vi "Swarm Method.vi"() -> ()   [LabVIEW 2014]
uses:
  <vilib>/Analysis/NI_AALPro.lvlib
  <vilib>/Analysis/baseanly.llb/Matrix Type of Inverse Matrix.ctl
  <vilib>/Analysis/NI_AALBase.lvlib
  <vilib>/Analysis/7linalg.llb/Solve Linear Equations (single right hand).vi
  Anchor/Anchor.lvclass
panel:
  in  "AnchorsArray":refnum<class "Anchor.lvclass">[](array[class])
  in  "Max bereik":dbl
  in  "d tags anchors":dbl[][](array[numeric])
  out "tag 3":i32
  in  "d tags onderling":dbl[](array[numeric])
  out "Solution Vector":dbl[](array[numeric]) format="%.2f"
  in  "Werkpunten":cluster{"a":dbl, "b":dbl}[](array[cluster])
  in  "# tags":i32=22
  out "tag 2":i32
  out "Tag 1":i32
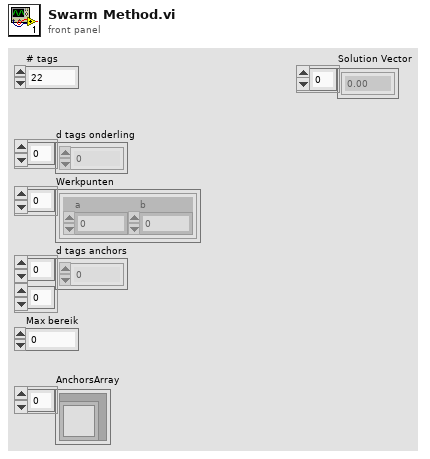
[diagram p1: front panel]
types:
  T1 = typedef "NI_AALBase.lvlib/Matrix Type of Inverse Matrix.ctl" = enum32{"General", "Positive Definite", "Lower Triangular", "Upper Triangular"}
  T2 = cluster{"Tag.lvclass":refnum<class "Tag.lvclass">, "Distance":dbl}[]
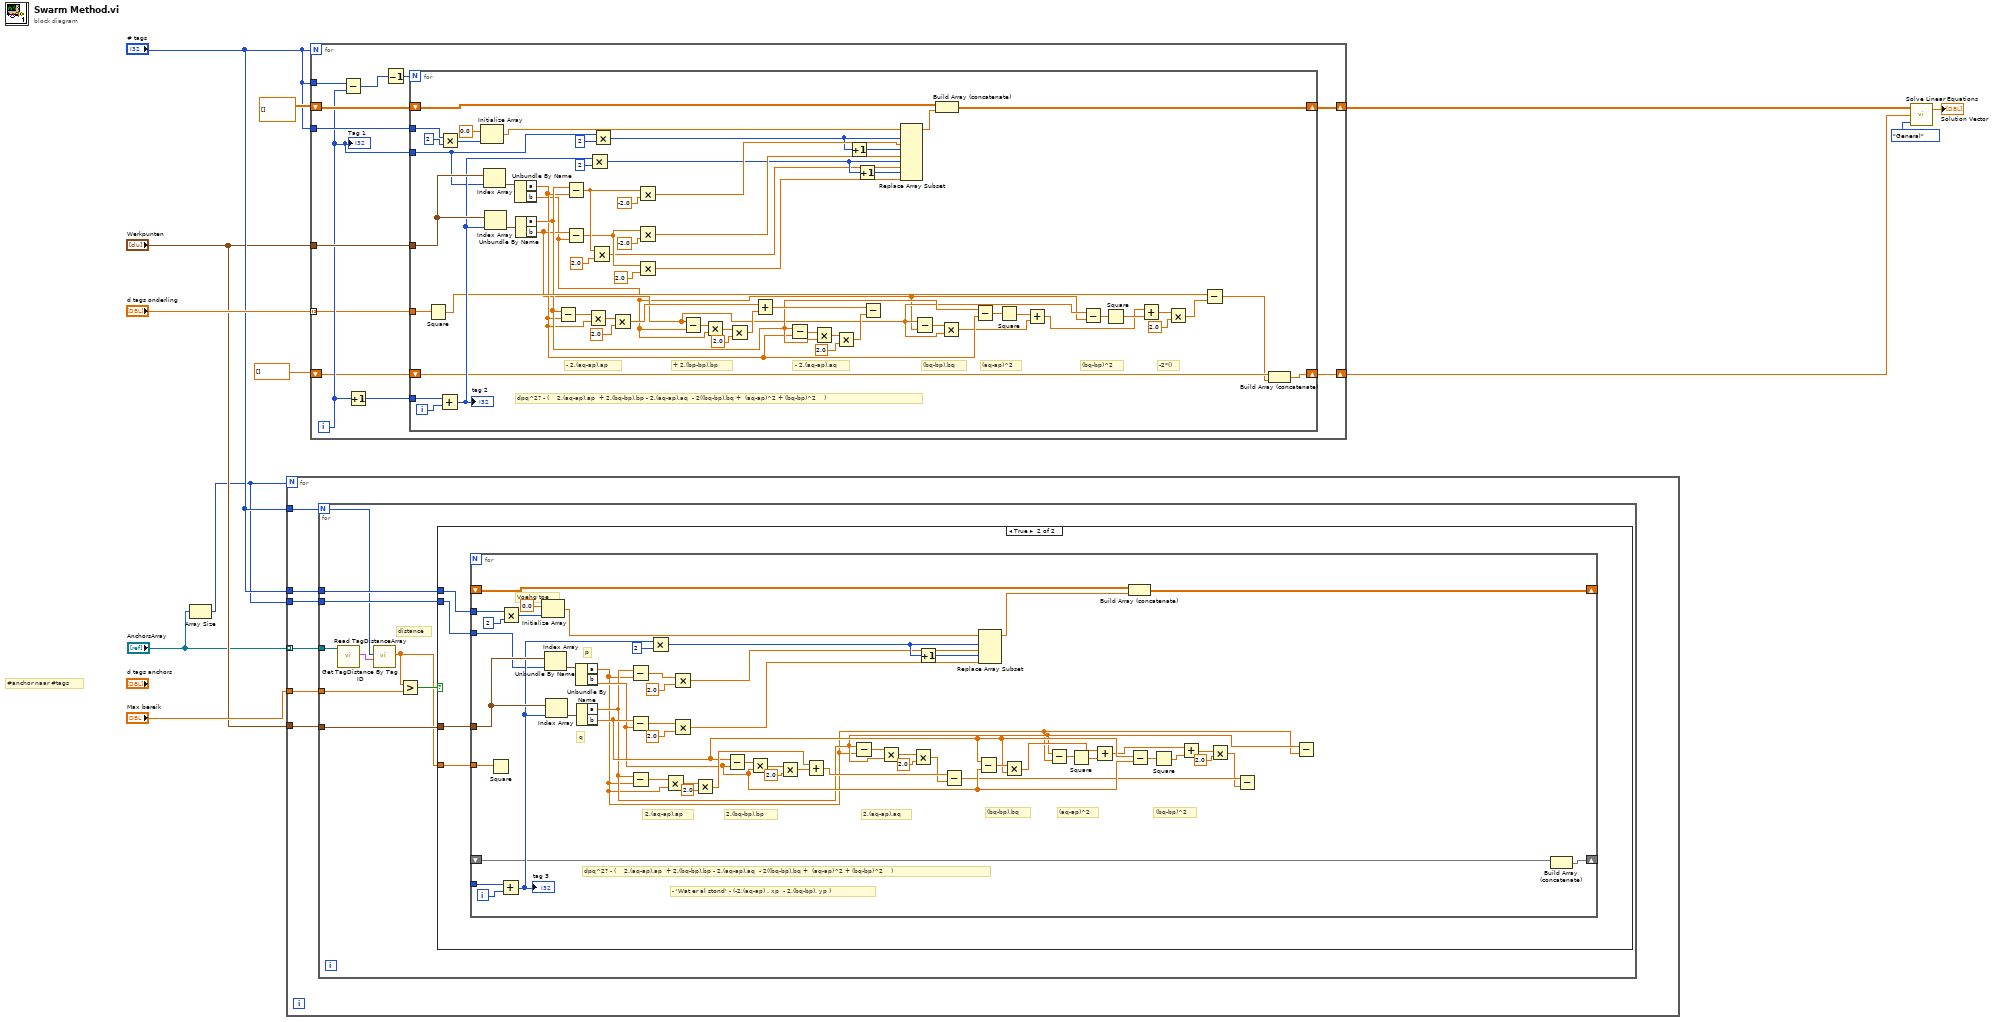
[diagram p0: block diagram]
diagram:
  # "#anchor naar #tags"
  n1 = Array Size(array="AnchorsArray") -> (size(s)=w1:i32)
  n2 = for {
    N: w1 -> [_]
    tunnel: "# tags" -> [w16]
    tunnel: "Max bereik" -> [w18]
    tunnel: "Werkpunten" -> [w17]
    tunnel: "# tags" -> [w15]
    tunnel: w1 -> [w14]
    tunnel: "AnchorsArray" -> [w13] mode=indexing
    n3 = for {
      N: w16 -> [w20]
      tunnel: w18 -> [w26]
      tunnel: w17 -> [w25]
      tunnel: w14 -> [w24]
      tunnel: w15 -> [w23]
      tunnel: w13 -> [w22]
      # "distance"
      n4 = call-dynamic "Read TagDistanceArray.vi"("Anchor in"=w22) -> ("TagDistanceArray"=w21:T2)  [unwired: 8 in, 2 out]
      n5 = call "Get TagDistance By Tag ID.vi"("TagDistanceArray"=w21, "TagID"=w20) -> ("Distance"=w19:dbl)  [unwired: 9 in]
      n6 = Greater?(x=w19, y=w26) -> (0:w27:bool)
      n7 = case shown="True" w27 {
        tunnel: w25 -> [_ w31]
        tunnel: w24 -> [_ w30]
        tunnel: w23 -> [_ w29]
        tunnel: w19 -> [_ w28]
        frame False {
        }
        frame True {
          # "Voehg toe"
          n8 = for {
            tunnel: _ -> [w85]
            shift-right: [w84] -> _
            shift-left: _ -> [w78]
            tunnel: w29 -> [w80]
            tunnel: w31 -> [w75]
            tunnel: w30 -> [w62]
            shift-right: [w61] -> _
            shift-left: _ -> [w63]
            tunnel: w28 -> [w60]
            i -> [w86]
            # "(bq-bp)^2"
            # "(aq-ap)^2"
            # "(bq-bp).bq"
            # "2.(aq-ap).aq"
            # "2.(bq-bp).bp"
            # "2.(aq-ap).ap"
            # "q"
            # "p"
            # "-\t'Wat er al stond' - (-2.(aq-ap) . xp  - 2.(bq-bp). yp )"
            # "dpq^2? - (    2.(aq-ap).ap  + 2.(bq-bp).bp - 2.(aq-ap).aq  - 2((bq-bp).bq +  (aq-ap)^2 + (bq-bp)^2    )"
            n9 = Square(x=w60) -> ()  [unwired: 1 out]
            n10 = Add(x=w85, y=w86) -> (x+y=w72:i32)
            "tag 3" <- w72
            n11 = Multiply(x=w80, y=2) -> (x*y=w83:i32)
            n12 = Initialize Array(0.0 ("element"), w83) -> (w77:dbl[])
            n13 = Index Array(array=w75, index=w62) -> (element=w76:cluster{"a":dbl, "b":dbl})
            n14 = Index Array(array=w75, index=w72) -> (element=w74:cluster{"a":dbl, "b":dbl})
            n15 = Unbundle By Name(w76) -> ("a"=w32:dbl, "b"=w41:dbl)
            n16 = Unbundle By Name(w74) -> ("a"=w33:dbl, "b"=w42:dbl)
            n17 = Subtract(x=w33, y=w32) -> (x-y=w67:dbl)
            n18 = Subtract(x=w42, y=w41) -> (x-y=w66:dbl)
            n19 = Subtract(x=w33, y=w32) -> (x-y=w59:dbl)
            n20 = Multiply(x=w72, y=2) -> (x*y=w71:i32)
            n21 = Multiply(x=w59, y=w32) -> (x*y=w58:dbl)
            n22 = Multiply(x=w67, y=2.0) -> (x*y=w65:dbl)
            n23 = Multiply(x=w66, y=2.0) -> (x*y=w64:dbl)
            n24 = Multiply(x=w58, y=2.0) -> (x*y=w53:dbl)
            n25 = Subtract(x=w42, y=w41) -> (x-y=w56:dbl)
            n26 = Multiply(x=w56, y=w41) -> (x*y=w55:dbl)
            n27 = Multiply(x=w55, y=2.0) -> (x*y=w52:dbl)
            n28 = Add(x=w53, y=w52) -> (x+y=w48:dbl)
            n29 = Subtract(x=w33, y=w32) -> (x-y=w51:dbl)
            n30 = Multiply(x=w51, y=w33) -> (x*y=w50:dbl)
            n31 = Multiply(x=w50, y=2.0) -> (x*y=w47:dbl)
            n32 = Increment(x=w71) -> (x+1=w70:i32)
            n33 = Subtract(x=w48, y=w47) -> (x-y=w35:dbl)
            n34 = Subtract(x=w42, y=w41) -> (x-y=w46:dbl)
            n35 = Replace Array Subset(array=w77, new element #1=w65, index #1=w71, new element #2=w64, index #2=w70) -> (w79:dbl[])
            n36 = Multiply(x=w46, y=w42) -> (x*y=w44:dbl)
            n37 = Subtract(x=w33, y=w32) -> (x-y=w45:dbl)
            n38 = Square(x=w45) -> (x^2=w43:dbl)
            n39 = Add(x=w44, y=w43) -> (x+y=w39:dbl)
            n40 = Build Array (concatenate)(w78, w79) -> (w84:dbl[][])
            n41 = Subtract(x=w42, y=w41) -> (x-y=w40:dbl)
            n42 = Square(x=w40) -> (x^2=w38:dbl)
            n43 = Add(x=w39, y=w38) -> (x+y=w37:dbl)
            n44 = Multiply(x=w37, y=2.0) -> (x*y=w34:dbl)
            n45 = Subtract(x=w35, y=w34) -> ()  [unwired: 1 out]
            n46 = Subtract(x=w33, y=w32) -> ()  [unwired: 1 out]
            n47 = Build Array (concatenate)(w63) -> (w61:void[])  [unwired: 1 in]
          }
        }
      }
    }
  }
  n48 = for {
    N: "# tags" -> [_]
    tunnel: "# tags" -> [w98]
    shift-right: [w93] -> w11
    shift-left: dbl[][] [] -> [w94]
    tunnel: "# tags" -> [w92]
    tunnel: "Werkpunten" -> [w91]
    shift-right: [w89] -> w9
    shift-left: dbl[] [] -> [w88]
    tunnel: "d tags onderling" -> [w87] mode=indexing
    i -> [w90]
    n49 = Subtract(x=w98, y=w90) -> (x-y=w97:i32)
    n50 = Increment(x=w90) -> (x+1=w95:i32)
    n51 = Decrement(x=w97) -> (x-1=w96:i32)
    n52 = for {
      N: w96 -> [_]
      tunnel: w95 -> [w160]
      shift-right: [w159] -> w93
      shift-left: w94 -> [w153]
      tunnel: w92 -> [w155]
      tunnel: w91 -> [w150]
      tunnel: w90 -> [w130]
      shift-right: [w129] -> w89
      shift-left: w88 -> [w131]
      tunnel: w87 -> [w128]
      i -> [w161]
      # "-2*()"
      # "(bq-bp)^2"
      # "(aq-ap)^2"
      # "(bq-bp).bq"
      # "- 2.(aq-ap).aq"
      # "+ 2.(bp-bp).bp"
      # "- 2.(aq-ap).ap"
      # "dpq^2? - (    2.(aq-ap).ap  + 2.(bq-bp).bp - 2.(aq-ap).aq  - 2((bq-bp).bq +  (aq-ap)^2 + (bq-bp)^2    )"
      n53 = Square(x=w128) -> (x^2=w127:dbl)
      n54 = Add(x=w160, y=w161) -> (x+y=w140:i32)
      "tag 2" <- w140
      n55 = Multiply(x=w155, y=2) -> (x*y=w158:i32)
      n56 = Initialize Array(0.0 ("element"), w158) -> (w152:dbl[])
      n57 = Index Array(array=w150, index=w130) -> (element=w151:cluster{"a":dbl, "b":dbl})
      n58 = Index Array(array=w150, index=w140) -> (element=w149:cluster{"a":dbl, "b":dbl})
      n59 = Unbundle By Name(w151) -> ("a"=w111:dbl, "b"=w106:dbl)
      n60 = Unbundle By Name(w149) -> ("a"=w112:dbl, "b"=w107:dbl)
      n61 = Subtract(x=w112, y=w111) -> (x-y=w125:dbl)
      n62 = Subtract(x=w112, y=w111) -> (x-y=w135:dbl)
      n63 = Subtract(x=w107, y=w106) -> (x-y=w134:dbl)
      n64 = Multiply(x=w125, y=w111) -> (x*y=w124:dbl)
      n65 = Multiply(x=w140, y=2) -> (x*y=w139:i32)
      n66 = Multiply(x=w135, y=2.0) -> (x*y=w133:dbl)
      n67 = Multiply(x=w130, y=2) -> (x*y=w143:i32)
      n68 = Multiply(x=w124, y=2.0) -> (x*y=w123:dbl)
      n69 = Multiply(x=w135, y=-2.0) -> (x*y=w146:dbl)
      n70 = Multiply(x=w134, y=-2.0) -> (x*y=w144:dbl)
      n71 = Multiply(x=w134, y=2.0) -> (x*y=w132:dbl)
      n72 = Subtract(x=w107, y=w106) -> (x-y=w122:dbl)
      n73 = Multiply(x=w122, y=w106) -> (x*y=w121:dbl)
      n74 = Multiply(x=w121, y=2.0) -> (x*y=w119:dbl)
      n75 = Add(x=w123, y=w119) -> (x+y=w115:dbl)
      n76 = Subtract(x=w112, y=w111) -> (x-y=w118:dbl)
      n77 = Multiply(x=w118, y=w112) -> (x*y=w117:dbl)
      n78 = Multiply(x=w117, y=2.0) -> (x*y=w114:dbl)
      n79 = Increment(x=w143) -> (x+1=w142:i32)
      n80 = Increment(x=w139) -> (x+1=w138:i32)
      n81 = Subtract(x=w115, y=w114) -> ()  [unwired: 1 out]
      n82 = Replace Array Subset(array=w152, new element #1=w146, index #1=w143, new element #2=w144, index #2=w142, new element #3=w133, index #3=w139, new element #4=w132, index #4=w138) -> (w154:dbl[])
      n83 = Subtract(x=w107, y=w106) -> (x-y=w113:dbl)
      n84 = Build Array (concatenate)(w153, w154) -> (w159:dbl[][])
      n85 = Multiply(x=w113, y=w107) -> (x*y=w108:dbl)
      n86 = Subtract(x=w112, y=w111) -> (x-y=w110:dbl)
      n87 = Square(x=w110) -> (x^2=w109:dbl)
      n88 = Add(x=w109, y=w108) -> (x+y=w103:dbl)
      n89 = Subtract(x=w107, y=w106) -> (x-y=w105:dbl)
      n90 = Square(x=w105) -> (x^2=w104:dbl)
      n91 = Add(x=w103, y=w104) -> (x+y=w102:dbl)
      n92 = Multiply(x=w102, y=2.0) -> (x*y=w100:dbl)
      n93 = Subtract(x=w127, y=w100) -> (x-y=w99:dbl)
      n94 = Build Array (concatenate)(w131, w99) -> (w129:dbl[])
    }
    "Tag 1" <- w90
  }
  n95 = call-poly <vilib>:"Solve Linear Equations.vi"("matrix type"=Matrix_Type_of_Inverse_Matrix."General", "Known Vector"=w9, "Input Matrix"=w11) -> ("Solution Vector"=→"Solution Vector":dbl[])  [unwired: 1 out]
